vi "DBC_Create_Status_Entries.vi"(4 "Config":T2={"Präfix"="", "Data Type"=1, "Number of Bits"=32} {"Data Type" items=["Signed", "Unsigned", "IEEE Float", "Byte Array"]}, 5 "Comment":T1[](array[typedef]), 6 "Optionsfelder":T3(ring), 7 "Name":T1[](array[typedef]), 8 "Fehler (Eingang, kein Fehler)":errorcluster, 9 "Scale":sgl[](array[numeric]), 10 "Frames":i32[](array[numeric]), 11 "Cluster (Eingang)":refnum<k21>) -> (0 "Fehler (Ausgang)":errorcluster, 3 "cluster out":refnum<k21>)   [LabVIEW 2020, in "CAN Konfig.lvlib"]
uses:
  CAN Konfig.lvlib
  Visualisierungs Elemente/String - Ausgabefeld.ctl
  SAE J-1939 SignalConfig.ctl
  <vilib>/xnet/xnet.llb/XNET Database Create (Frame).vi
  <resource>/objmgr/xnet.rc
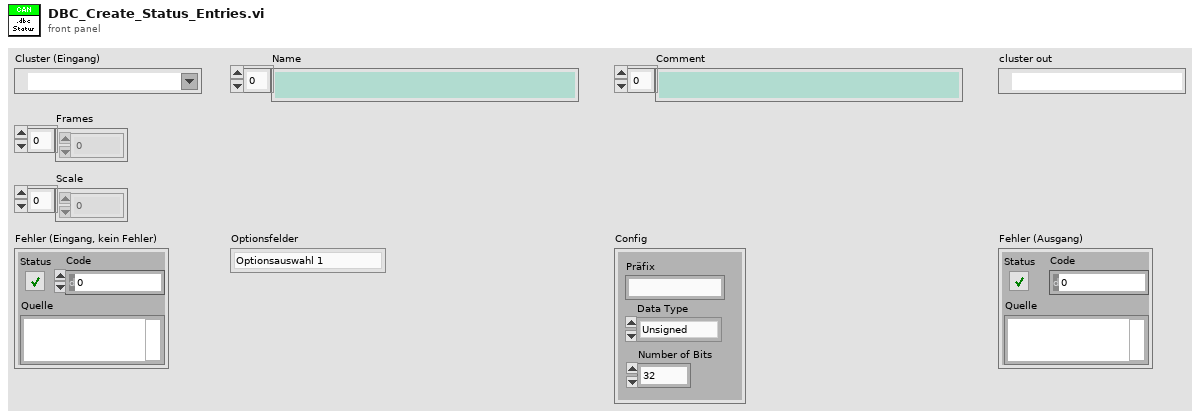
[diagram p1: front panel]
types:
  T1 = typedef "String - Ausgabefeld.ctl" = string
  T2 = cluster{"Präfix":string, "Data Type":u32, "Number of Bits":u32}
  T3 = enum32{"Optionsauswahl 1", "Optionsauswahl 2", "Optionsauswahl 3"}
  T4 = typedef "CAN Konfig.lvlib/SAE J-1939 SignalConfig.ctl" = cluster{"Index":i32, "Start Bit":u32, "Data Type":u32, "Number of Bits":u32}
  T5 = cluster{"String - Ausgabefeld":T1, "String - Ausgabefeld":T1}
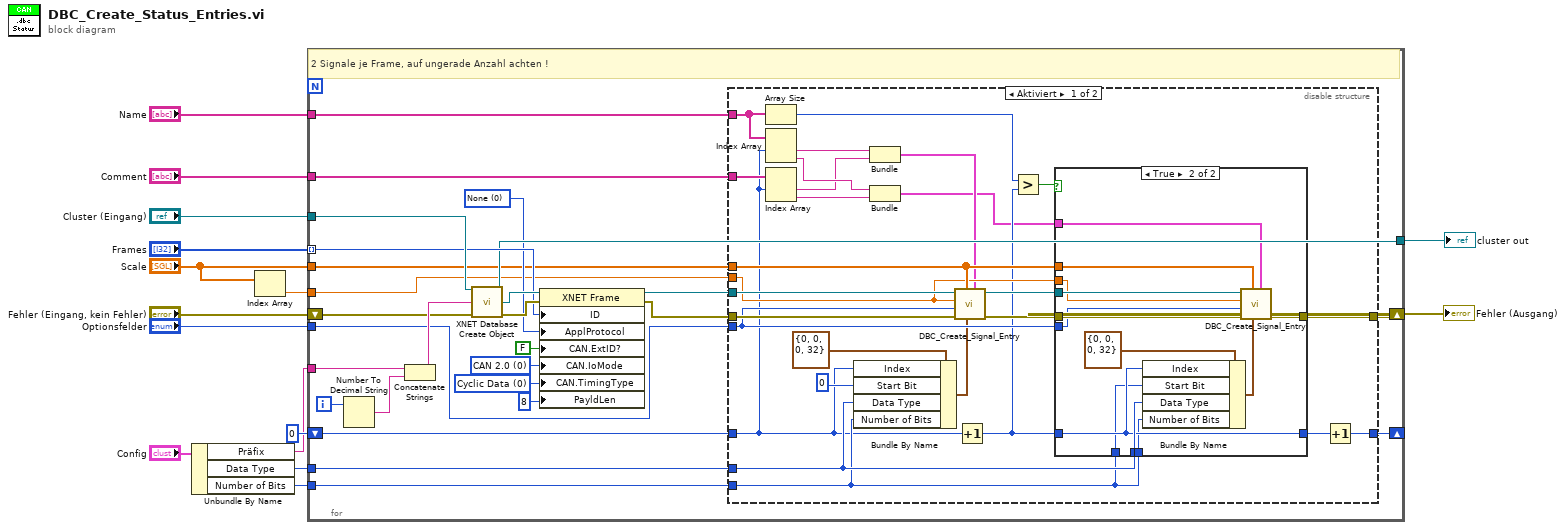
[diagram p0: block diagram]
diagram:
  n1 = Unbundle By Name("Config") -> ("Präfix"=w4:string, "Data Type"=w3:u32, "Number of Bits"=w2:u32)
  n2 = Index Array(array="Scale") -> (element=w14:sgl)  [unwired: 1 in]
  n3 = for {
    tunnel: "Frames" -> [w35] mode=indexing
    tunnel: "Name" -> [w24]
    tunnel: "Scale" -> [w28]
    tunnel: "Optionsfelder" -> [w25]
    tunnel: "Cluster (Eingang)" -> [w42]
    tunnel: w14 -> [w27]
    shift-right: [w29] -> w15
    shift-left: "Fehler (Eingang, kein Fehler)" -> [w33]
    tunnel: [w34] -> w7
    shift-right: [w26] -> _
    shift-left: 0 -> [w30]
    tunnel: w4 -> [w19]
    tunnel: w3 -> [w18]
    tunnel: w2 -> [w17]
    tunnel: "Comment" -> [w16]
    i -> [w31]
    w21 = u32 0 items=["Cyclic Data", "Event Data", "Cyclic Remote", "Event Remote", "Cyclic/Event"] ("CAN:Timing Type")
    w22 = u32 0 items=["CAN 2.0", "CAN FD", "CAN FD+BRS"] ("CAN:I/O Mode")
    w32 = u32 0 items=["None", "J1939"] ("Application Protocol")
    # "2 Signale je Frame, auf ungerade Anzahl achten !"
    n4 = Number To Decimal String(number=w31) -> (decimal integer string=w40:string)  [unwired: 1 in]
    n5 = Concatenate Strings(w19, w40) -> (w41:string)
    n6 = call-poly <vilib>:"XNET Database Create Object.vi"("cluster in"=w42, "frame name"=w41, "error in (no error)"=w33) -> ("cluster out"=w34:refnum<k21>, "frame out"=w39:refnum<k21>, "error out"=w37:errorcluster)  [unwired: 10 in]
    n7 = property class="XNET Frame"(reference=w39, error in=w37, "ID"=w35, "ApplProtocol"=w32, "CAN.ExtID?"=FALSE ("CAN:Extended Identifier?"), "CAN.IoMode"=w22, "CAN.TimingType"=w21, "PayldLen"=u32 8 ("Payload Length")) -> (reference out=w38:refnum<k21>, error out=w36:errorcluster)
    n8 = disable-structure shown="Aktiviert" {
      disable-tunnel: w38 -> [w69 _]
      disable-tunnel: w36 -> [w68 w85]
      disable-tunnel: w30 -> [w48 _]
      disable-tunnel: [w65 w85] -> w29
      disable-tunnel: w28 -> [w63 _]
      disable-tunnel: w27 -> [w62 _]
      disable-tunnel: [w61 _] -> w26
      disable-tunnel: w25 -> [w60 _]
      disable-tunnel: w24 -> [w57 _]
      disable-tunnel: w18 -> [w52 _]
      disable-tunnel: w17 -> [w50 _]
      disable-tunnel: w16 -> [w49 _]
      frame Enabled {
        n9 = Array Size(array=w57) -> (size(s)=w55:i32)
        n10 = Index Array(array=w57, index #1=w48) -> (element #1=w47:T1, element #2=w64:T1)  [unwired: 1 in]
        n11 = Index Array(array=w49, index #1=w48) -> (element #1=w46:T1, element #2=w43:T1)  [unwired: 1 in]
        n12 = Bundle By Name(cluster=T4 {"Index"=0, "Start Bit"=0, "Data Type"=0, "Number of Bits"=32} ("Config"), "Index"=w48, "Start Bit"=u32 0, "Data Type"=w52, "Number of Bits"=w50) -> (w58:T4)
        n13 = Bundle("String - Ausgabefeld"=w47, "String - Ausgabefeld"=w46) -> (w45:T5)  [unwired: 1 in]
        n14 = Bundle("String - Ausgabefeld"=w64, "String - Ausgabefeld"=w43) -> (w44:T5)  [unwired: 1 in]
        n15 = call "DBC_Create_Signal_Entry.vi"("Name Cluster"=w45, "Config"=w58, "Status Scale"=w63, "Fehler (Eingang, kein Fehler)"=w68, "Optionsfelder Status"=w60, "Scale overall"=w62, "Frame (Eingang)"=w69) -> ("Fehler (Ausgang)"=w66:errorcluster, "Referenz (Ausgang)"=w67:refnum<k21>)  [unwired: 2 in, 1 out]
        n16 = Increment(x=w48) -> (x+1=w54:i32)
        n17 = Greater?(x=w55, y=w54) -> (0:w56:bool)
        n18 = case shown="True" w56 {
          tunnel: w67 -> [_ w84]
          tunnel: w66 -> [w71 w83]
          tunnel: [w71 w82] -> w65
          tunnel: w44 -> [_ w81]
          tunnel: w63 -> [_ w80]
          tunnel: w62 -> [_ w79]
          tunnel: w60 -> [_ w78]
          tunnel: w54 -> [w70 w75]
          tunnel: w52 -> [_ w77]
          tunnel: [w70 w75] -> w53
          tunnel: w50 -> [_ w73]
          tunnel: w50 -> [_ w72]
          frame False {
          }
          frame True {
            n19 = Bundle By Name(cluster=T4 {"Index"=0, "Start Bit"=0, "Data Type"=0, "Number of Bits"=32} ("Config"), "Index"=w75, "Start Bit"=w72, "Data Type"=w77, "Number of Bits"=w73) -> (w76:T4)
            n20 = call "DBC_Create_Signal_Entry.vi"("Name Cluster"=w81, "Config"=w76, "Status Scale"=w80, "Fehler (Eingang, kein Fehler)"=w83, "Optionsfelder Status"=w78, "Scale overall"=w79, "Frame (Eingang)"=w84) -> ("Fehler (Ausgang)"=w82:errorcluster)  [unwired: 2 in, 2 out]
          }
        }
        n21 = Increment(x=w53) -> (x+1=w61:i32)
      }
      frame Disabled {
      }
    }
  }
  "Fehler (Ausgang)" <- w15
  "cluster out" <- w7
